vi "JoyScaleTank2.vi"(8 "Tolerance":dbl, 10 "x Axis":dbl(slide) scale=-127.0..127.0, 11 "y Axis":dbl(slide) scale=-127.0..127.0 scale format="%#_4g") -> (1 "Speed Right":dbl(knob) scale=-1.0..1.0, 2 "Speed Left":dbl(knob) scale=-1.0..1.0, 3 "Speed":dbl(knob) scale=-1.0..1.0)   [LabVIEW 2011]
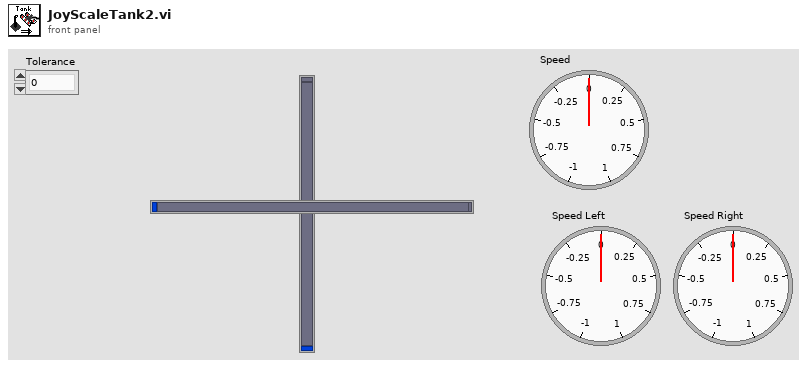
[diagram p1: front panel]
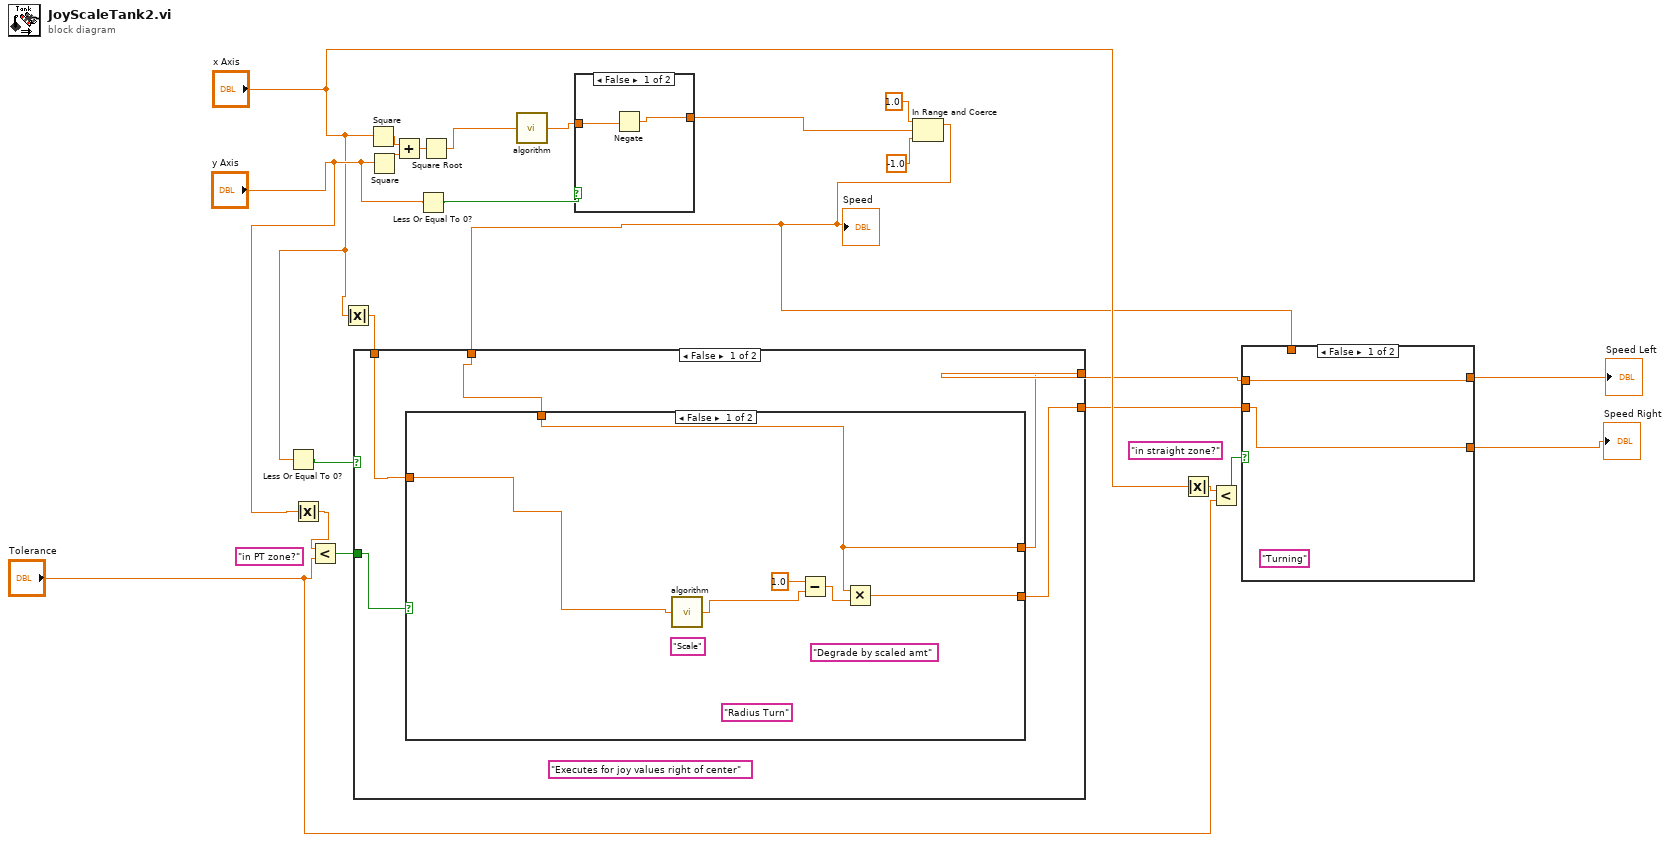
[diagram p0: block diagram]
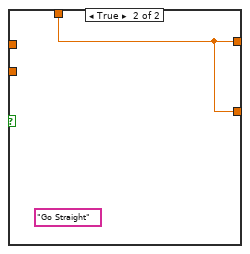
[diagram p2: hidden frame]
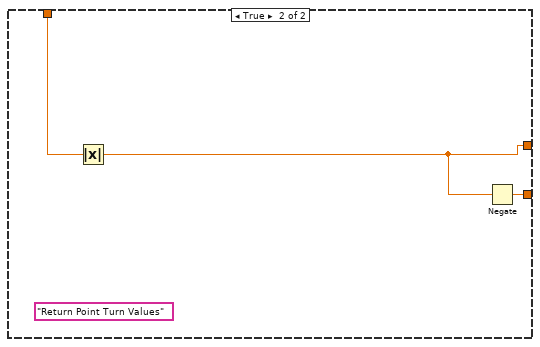
[diagram p3: hidden frame]
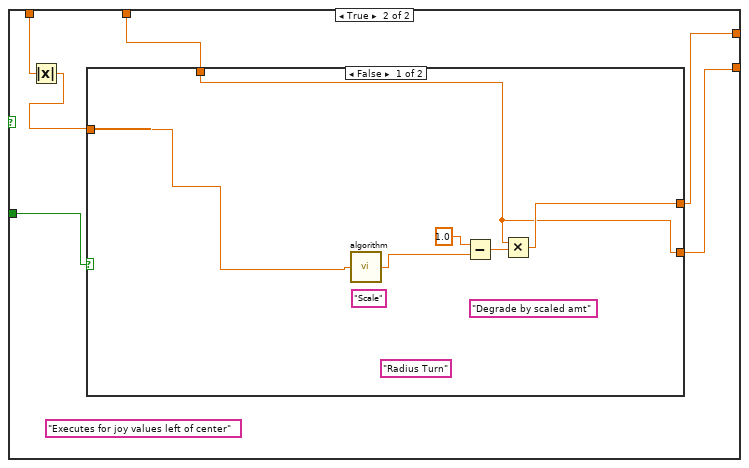
[diagram p4: hidden frame]
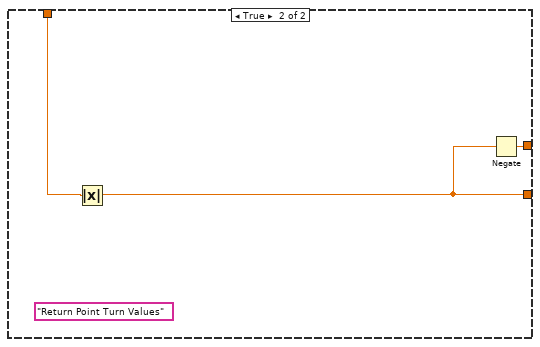
[diagram p5: hidden frame]
diagram:
  (unwired) "in straight zone?"
  (unwired) "in PT zone?"
  n1 = Less Or Equal To 0?(x="x Axis") -> (x <= 0?=w20:bool)
  n2 = Absolute Value(x="y Axis") -> (abs(x)=w11:dbl)
  n3 = Less?(x=w11, y="Tolerance") -> (x < y?=w10:bool)
  n4 = Absolute Value(x="x Axis") -> (abs(x)=w12:dbl)
  n5 = Square(x="x Axis") -> (x^2=w21:dbl)
  n6 = Square(x="y Axis") -> (x^2=w22:dbl)
  n7 = Add(x=w21, y=w22) -> (x+y=w23:dbl)
  n8 = Less Or Equal To 0?(x="y Axis") -> (x <= 0?=w17:bool)
  n9 = Square Root(x=w23) -> (sqrt(x)=w16:dbl)
  n10 = call "algorithm.vi"("x"=w16) -> ("f(x)"=w15:dbl)
  n11 = case shown="False" w17 {
    tunnel: [w24 w26] -> w14
    tunnel: w15 -> [w25 w26]
    frame False {
      n12 = Negate(x=w25) -> (-x=w24:dbl)
    }
    frame True {
    }
  }
  n13 = In Range and Coerce(upper limit=1.0, x=w14, lower limit=-1.0) -> (coerced(x)=w2:dbl)  [unwired: 1 out]
  "Speed" <- w2
  n14 = case shown="False" w20 {
    tunnel: [w30 w46] -> w5
    tunnel: w12 -> [w29 w43]
    tunnel: w2 -> [w28 w44]
    tunnel: [w31 w45] -> w4
    tunnel: w10 -> [w27 w41]
    frame False {
      (unwired) "Executes for joy values right of center"
      n15 = case shown="False" w27 {
        tunnel: [w37 w39] -> w30
        tunnel: [w36 w38] -> w31
        tunnel: w28 -> [w36 w40]
        tunnel: w29 -> [w32 _]
        frame False {
          (unwired) "Radius Turn"
          (unwired) "Degrade by scaled amt"
          (unwired) "Scale"
          n16 = call "algorithm.vi"("x"=w32) -> ("f(x)"=w35:dbl)
          n17 = Subtract(x=1.0, y=w35) -> (x-y=w34:dbl)
          n18 = Multiply(x=w36, y=w34) -> (x*y=w37:dbl)
        }
        frame True {
          (unwired) "Return Point Turn Values"
          n19 = Absolute Value(x=w40) -> (abs(x)=w38:dbl)
          n20 = Negate(x=w38) -> (-x=w39:dbl)
        }
      }
    }
    frame True {
      (unwired) "Executes for joy values left of center"
      n21 = Absolute Value(x=w43) -> (abs(x)=w42:dbl)
      n22 = case shown="False" w41 {
        tunnel: [w51 w53] -> w46
        tunnel: [w52 w55] -> w45
        tunnel: w44 -> [w51 w54]
        tunnel: w42 -> [w47 _]
        frame False {
          (unwired) "Radius Turn"
          (unwired) "Degrade by scaled amt"
          (unwired) "Scale"
          n23 = call "algorithm.vi"("x"=w47) -> ("f(x)"=w50:dbl)
          n24 = Subtract(x=1.0, y=w50) -> (x-y=w49:dbl)
          n25 = Multiply(x=w51, y=w49) -> (x*y=w52:dbl)
        }
        frame True {
          (unwired) "Return Point Turn Values"
          n26 = Absolute Value(x=w54) -> (abs(x)=w53:dbl)
          n27 = Negate(x=w53) -> (-x=w55:dbl)
        }
      }
    }
  }
  n28 = Absolute Value(x="x Axis") -> (abs(x)=w9:dbl)
  n29 = Less?(x=w9, y="Tolerance") -> (x < y?=w6:bool)
  n30 = case shown="False" w6 {
    tunnel: w4 -> [w57 _]
    tunnel: w5 -> [w56 _]
    tunnel: [w57 w58] -> w3
    tunnel: w2 -> [_ w58]
    tunnel: [w56 w58] -> w1
    frame False {
      (unwired) "Turning"
    }
    frame True {
      (unwired) "Go Straight"
    }
  }
  "Speed Left" <- w3
  "Speed Right" <- w1
